vi "MLPClassifier.vi"(8 "error in":errorcluster) -> (0 "error out":errorcluster, 3 "out":refnum<class "MLPClassifier.lvclass">)   [LabVIEW 2020]
doc: "Multi-layer Perceptron classifier.\n\n This model optimizes the log-loss function using LBFGS or stochastic\n gradient descent.\n\n .. versionadded:: 0.18\n\n Parameters\n ----------\n hidden_layer_sizes : tuple, length = n_layers - 2, default=(100,)\n The ith element represents the number of neurons in the ith\n hidden layer.\n\n activation : {'identity', 'logistic', 'tanh', 'relu'}, default='relu'\n Activation function for the hidden layer.\n\n - 'identity', no-op activation, useful to implement linear bottleneck,\n returns f(x) = x\n\n - 'logistic', the logistic sigmoid function,\n returns f(x) = 1 / (1 + exp(-x)).\n\n - 'tanh', the hyperbolic tan function,\n returns f(x) = tanh(x).\n\n - 'relu', the rectified linear unit function,\n returns f(x) = max(0, x)\n\n solver : {'lbfgs', 'sgd', 'adam'}, default='adam'\n The solver for weight optimization.\n\n - 'lbfgs' is an optimizer in the family of quasi-Newton methods.\n\n - 'sgd' refers to stochastic gradient descent.\n\n - 'adam' refers to a stochastic gradient-based optimizer proposed\n by Kingma, Diederik, and Jimmy Ba\n\n Note: The default solver 'adam' works pretty well on relatively\n large datasets (with thousands of training samples or more) in terms of\n both training time and validation score.\n For small datasets, however, 'lbfgs' can converge faster and perform\n better.\n\n alpha : float, default=0.0001\n L2 penalty (regularization term) parameter.\n\n batch_size : int, default='auto'\n Size of minibatches for stochastic optimizers.\n If the solver is 'lbfgs', the classifier will not use minibatch.\n When set to \"auto\", `batch_size=min(200, n_samples)`\n\n learning_rate : {'constant', 'invscaling', 'adaptive'}, default='constant'\n Learning rate schedule for weight updates.\n\n - 'constant' is a constant learning rate given by\n 'learning_rate_init'.\n\n - 'invscaling' gradually decreases the learning rate at each\n time step 't' using an inverse scaling exponent of 'power_t'.\n effective_learning_rate = learning_rate_init / pow(t, power_t)\n\n - 'adaptive' keeps the learning rate constant to\n 'learning_rate_init' as long as training loss keeps decreasing.\n Each time two consecutive epochs fail to decrease training loss by at\n least tol, or fail to increase validation score by at least tol if\n 'early_stopping' is on, the current learning rate is divided by 5.\n\n Only used when ``solver='sgd'``.\n\n learning_rate_init : double, default=0.001\n The initial learning rate used. It controls the step-size\n in updating the weights. Only used when solver='sgd' or 'adam'.\n\n power_t : double, default=0.5\n The exponent for inverse scaling learning rate.\n It is used in updating effective learning rate when the learning_rate\n is set to 'invscaling'. Only used when solver='sgd'.\n\n max_iter : int, default=200\n Maximum number of iterations. The solver iterates until convergence\n (determined by 'tol') or this number of iterations. For stochastic\n solvers ('sgd', 'adam'), note that this determines the number of epochs\n (how many times each data point will be used), not the number of\n gradient steps.\n\n shuffle : bool, default=True\n Whether to shuffle samples in each iteration. Only used when\n solver='sgd' or 'adam'.\n\n random_state : int, RandomState instance, default=None\n Determines random number generation for weights and bias\n initialization, train-test split if early stopping is used, and batch\n sampling when solver='sgd' or 'adam'.\n Pass an int for reproducible results across multiple function calls.\n See :term:`Glossary <random_state>`.\n\n tol : float, default=1e-4\n Tolerance for the optimization. When the loss or score is not improving\n by at least ``tol`` for ``n_iter_no_change`` consecutive iterations,\n unless ``learning_rate`` is set to 'adaptive', convergence is\n considered to be reached and training stops.\n\n verbose : bool, default=False\n Whether to print progress messages to stdout.\n\n warm_start : bool, default=False\n When set to True, reuse the solution of the previous\n call to fit as initialization, otherwise, just erase the\n previous solution. See :term:`the Glossary <warm_start>`.\n\n momentum : float, default=0.9\n Momentum for gradient descent update. Should be between 0 and 1. Only\n used when solver='sgd'.\n\n nesterovs_momentum : bool, default=True\n Whether to use Nesterov's momentum. Only used when solver='sgd' and\n momentum > 0.\n\n early_stopping : bool, default=False\n Whether to use early stopping to terminate training when validation\n score is not improving. If set to true, it will automatically set\n aside 10% of training data as validation and terminate training when\n validation score is not improving by at least tol for\n ``n_iter_no_change`` consecutive epochs. The split is stratified,\n except in a multilabel setting.\n If early stopping is False, then the training stops when the training\n loss does not improve by more than tol for n_iter_no_change consecutive\n passes over the training set.\n Only effective when solver='sgd' or 'adam'\n\n validation_fraction : float, default=0.1\n The proportion of training data to set aside as validation set for\n early stopping. Must be between 0 and 1.\n Only used if early_stopping is True\n\n beta_1 : float, default=0.9\n Exponential decay rate for estimates of first moment vector in adam,\n should be in [0, 1). Only used when solver='adam'\n\n beta_2 : float, default=0.999\n Exponential decay rate for estimates of second moment vector in adam,\n should be in [0, 1). Only used when solver='adam'\n\n epsilon : float, default=1e-8\n Value for numerical stability in adam. Only used when solver='adam'\n\n n_iter_no_change : int, default=10\n Maximum number of epochs to not meet ``tol`` improvement.\n Only effective when solver='sgd' or 'adam'\n\n .. versionadded:: 0.20\n\n max_fun : int, default=15000\n Only used when solver='lbfgs'. Maximum number of loss function calls.\n The solver iterates until convergence (determined by 'tol'), number\n of iterations reaches max_iter, or this number of loss function calls.\n Note that number of loss function calls will be greater than or equal\n to the number of iterations for the `MLPClassifier`.\n\n .. versionadded:: 0.22\n\n Attributes\n ----------\n classes_ : ndarray or list of ndarray of shape (n_classes,)\n Class labels for each output.\n\n loss_ : float\n The current loss computed with the loss function.\n\n best_loss_ : float\n The minimum loss reached by the solver throughout fitting.\n\n loss_curve_ : list of shape (`n_iter_`,)\n The ith element in the list represents the loss at the ith iteration.\n\n t_ : int\n The number of training samples seen by the solver during fitting.\n\n coefs_ : list of shape (n_layers - 1,)\n The ith element in the list represents the weight matrix corresponding\n to layer i.\n\n intercepts_ : list of shape (n_layers - 1,)\n The ith element in the list represents the bias vector corresponding to\n layer i + 1.\n\n n_iter_ : int\n The number of iterations the solver has run.\n\n n_layers_ : int\n Number of layers.\n\n n_outputs_ : int\n Number of outputs.\n\n out_activation_ : str\n Name of the output activation function.\n\n \nAvailable methods:\nFit\nPredict\nScore\nGet Attributes\nGet Params\nSet Params"
uses:
  MultiLayerPerceptron/MLPClassifier/MLPClassifier.lvclass
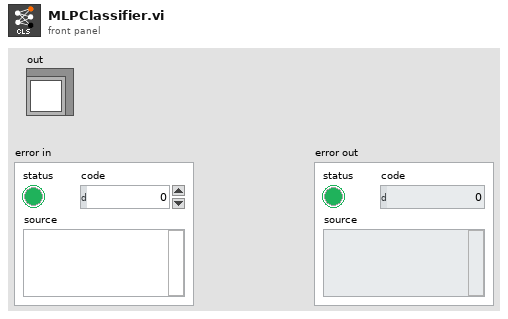
[diagram p1: front panel]
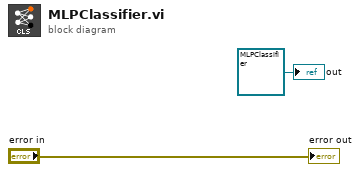
[diagram p0: block diagram]
diagram:
  "out" <- refnum<class "MLPClassifier.lvclass"> refnum ("model")
  "error out" <- "error in"
